vi "check if subpanel should be closed.vi"(8 "error in":errorcluster, 10 "SubPanel in":refnum<vi>, 11 "node in":T1) -> (0 "error out":errorcluster, 2 "needs closing":bool, 3 "node out":T1)   [LabVIEW 2013, in "Standard Editor.lvlib"]
uses:
  Standard Editor.lvlib
  <vilib>/NI/CEF/CEF_TreeControl/Node/NodeRef.ctl
  <vilib>/NI/CEF/CEF_TreeControl/Node/NISE_CEF_Node.lvclass
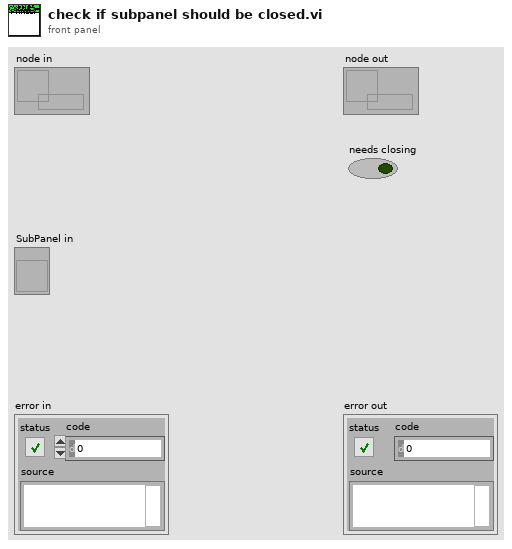
[diagram p1: front panel]
types:
  T1 = typedef "NISE_CEF_Node.lvclass/NodeRef.ctl" = refnum<data-value>
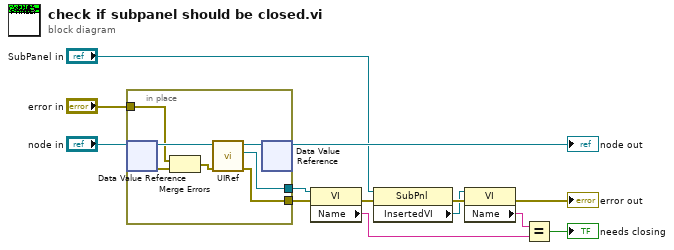
[diagram p0: block diagram]
diagram:
  n1 = in-place {
    in-place-border: "error in" -> [w17]
    in-place-border: [w18] -> w10
    in-place-border: [w16] -> w9
    n2 = in-place-dvr #1("node in") -> (w20:refnum<class "NISE_CEF_Node.lvclass">, w14:errorcluster)
    n3 = Merge Errors(w17, w14) -> (w15:errorcluster)
    n4 = call-dynamic "UIRef.vi"("error in"=w15, "node in"=w20) -> ("error out"=w16:errorcluster, "VI refnum"=w18:refnum<vi>, "node out"=w19:refnum<class "NISE_CEF_Node.lvclass">)  [unwired: 7 in]
    n5 = in-place-dvr #1(w19) -> (→"node out":T1)  [unwired: 1 out]
  }
  n6 = property class="VI"(reference=w10, error in=w9) -> (error out=w5:errorcluster, "Name"=w2:string)  [unwired: 1 out]
  n7 = property class="SubPnl"(reference="SubPanel in", error in=w5) -> (error out=w7:errorcluster, "InsertedVI"=w6:refnum<vi>)  [unwired: 1 out]
  n8 = property class="VI"(reference=w6, error in=w7) -> (error out=→"error out":errorcluster, "Name"=w3:string)  [unwired: 1 out]
  n9 = Equal?(x=w3, y=w2) -> (x = y?=→"needs closing":bool)
